vi "Get All Sinks.vi"(8 "error in (no error)":errorcluster, 11 "Sink Look Up Table in":refnum<class "Sink Look Up Table.lvclass">) -> (0 "error out":errorcluster, 1 "Names":string[](array[string]), 2 "Sinks":refnum<data-value>[](array[refnum]), 3 "Sink Look Up Table out":refnum<class "Sink Look Up Table.lvclass">)   [LabVIEW 2016, in "Stream Log.lvlib" / "Sink Look Up Table.lvclass"]
doc: "--\nCopyright © 2017 Composed SystemsI All rights reserved.\n\nAuthor: Jon McBee <jon.mcbee@composed.io>\n\nThis library is provided \"AS IS\" ,WITHOUT WARRANTIES OR\nCONDITIONS OF ANY KIND, either express or implied.\n\nComposed Systems -- composed.io\n\nStream 0.0.1.1\nJon McBee - Composed Systems\nCopyright (c) 2017, Composed Systems"
uses:
  <userlib>/Composed Systems/Stream/Log/Sink Look Up Table/Sink Look Up Table.lvclass
  C:/Program Files (x86)/National Instruments/LabVIEW 2016/user.lib/Composed Systems/Stream/Look Up Table/Look Up Table/Look Up Table.lvclass
  <userlib>/Composed Systems/Stream/Log/Log Sink/Log Sink.lvclass
  <userlib>/Composed Systems/Stream/Look Up Table/Look Up Table/Look Up Table.lvclass
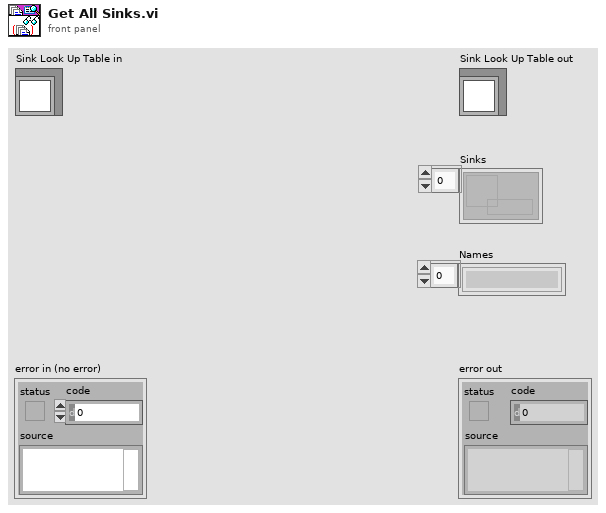
[diagram p1: front panel]
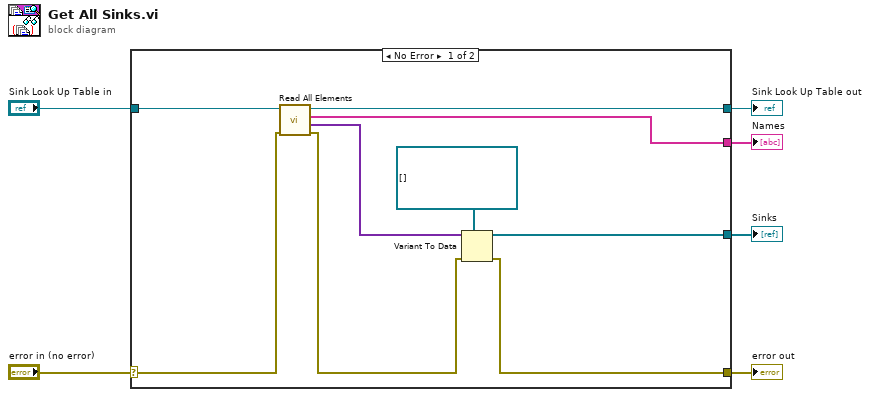
[diagram p0: block diagram]
diagram:
  n1 = case shown="No Error" "error in (no error)" {
    selector: "error in (no error)" -> [w10 w17]
    tunnel: [w8 w17] -> w5
    tunnel: [w14 w16] -> w3
    tunnel: "Sink Look Up Table in" -> [w15 w16]
    tunnel: [w12 _] -> w2
    tunnel: [w7 _] -> w1
    frame No Error {
      n2 = call <userlib>:"Read All Elements.vi"("error in (no error)"=w10, "Look Up Table in"=w15) -> ("error out"=w9:errorcluster, "All Elements"=w13:variant[], "Names"=w12:string[], "Look Up Table out"=w14:refnum<class "Sink Look Up Table.lvclass">)  [unwired: 6 in]
      n3 = Variant To Data(error in=w9, type=refnum<data-value>[] [], Variant=w13) -> (data=w7:refnum<data-value>[], error out=w8:errorcluster)
    }
    frame Error {
    }
  }
  "error out" <- w5
  "Sink Look Up Table out" <- w3
  "Names" <- w2
  "Sinks" <- w1
